vi "UpdateSwitches.vi"(8 "error in (no error)":errorcluster, 11 "SnakeGame in":refnum<class "SnakeGame.lvclass">) -> (0 "error out":errorcluster, 3 "SnakeGame out":refnum<class "SnakeGame.lvclass">)   [LabVIEW 2019, in "RT_Game.lvlib" / "SnakeGame.lvclass"]
uses:
  SnakeGame.lvclass
  SnakeGame.lvclass/SnakeGame.ctl
  GameObject/GameObject.lvclass/GameObject.ctl
  GameObject/Read IsActive.vi
  PongSwitch/SnakeSwitch.lvclass
  C:/Users/FreshBob/Dropbox/VIs/myRIO_GameConsole/RT/RT_Game/GameObject/GameObject.lvclass
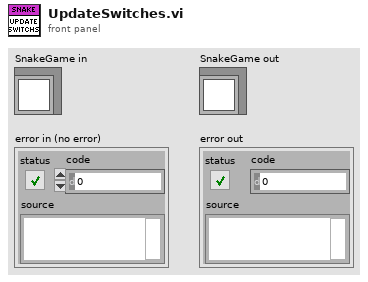
[diagram p1: front panel]
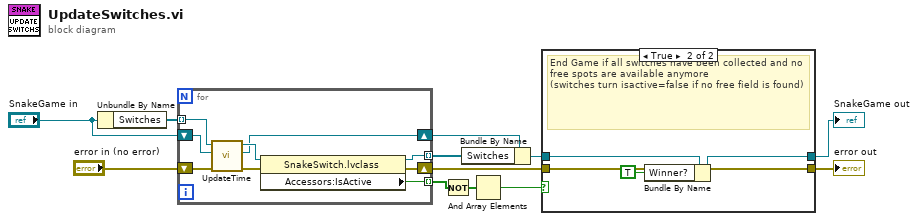
[diagram p0: block diagram]
diagram:
  n1 = Unbundle By Name("SnakeGame in") -> ("Switches"=w9:refnum<class "SnakeSwitch.lvclass">[])
  n2 = for {
    tunnel: w9 -> [w19] mode=indexing
    tunnel: [w16] -> w10 mode=indexing
    shift-right: [w18] -> w11
    shift-left: "error in (no error)" -> [w21]
    tunnel: [w15] -> w8 mode=indexing
    shift-right: [w14] -> w2
    shift-left: "SnakeGame in" -> [w13]
    n3 = call "UpdateTime.vi"("error in (no error)"=w21, "SnakeGame in"=w13, "SnakeSwitch in"=w19) -> ("error out"=w20:errorcluster, "SnakeGame out"=w14:refnum<class "SnakeGame.lvclass">, "SnakeSwitch out"=w17:refnum<class "SnakeSwitch.lvclass">)  [unwired: 6 in]
    n4 = property class="SnakeSwitch.lvclass"(reference=w17, error in=w20) -> (reference out=w16:refnum<class "SnakeSwitch.lvclass">, error out=w18:errorcluster, "Accessors:IsActive"=w15:bool)
  }
  n5 = Not(x=w8) -> (.not. x?=w1:bool[])
  n6 = Bundle By Name(cluster=w2, "Switches"=w10) -> (w6:refnum<class "SnakeGame.lvclass">)
  n7 = And Array Elements(Boolean array=w1) -> (logical AND=w4:bool)
  n8 = case shown="True" w4 {
    tunnel: w11 -> [w22 w27]
    tunnel: [w22 w27] -> w7
    tunnel: w6 -> [w23 w26]
    tunnel: [w23 w25] -> w5
    frame False {
    }
    frame True {
      # "End Game if all switches have been collected and no free spots are available anymore\n(switches turn isactive=false if no free field is found)"
      n9 = Bundle By Name(cluster=w26, "Winner?"=TRUE) -> (w25:refnum<class "SnakeGame.lvclass">)
    }
  }
  "error out" <- w7
  "SnakeGame out" <- w5
